vi "Open OCR Session.vi"() -> (0 "error out":errorcluster, 3 "IMAQ OCR Session":T1)   [LabVIEW 2011]
uses:
  <vilib>/vision/OCR.llb/IMAQ OCR Session.ctl
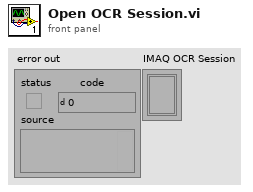
[diagram p1: front panel]
types:
  T1 = typedef "IMAQ OCR Session.ctl" = refnum<k1>
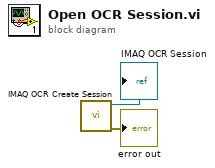
[diagram p0: block diagram]
diagram:
  n1 = call "IMAQ OCR Create Session"() -> ("error out"=→"error out":errorcluster, "IMAQ OCR Session"=→"IMAQ OCR Session":T1)  [unwired: 10 in]
